vi "LogLabVIEWError.vi"(8 "Error in (no error)":errorcluster, 10 "Error in":errorcluster, 11 "Log in":refnum<class "Log.lvclass">) -> (0 "Error out":errorcluster, 3 "Log out":refnum<class "Log.lvclass">)   [LabVIEW 2011, in "Log.lvclass"]
uses:
  Log.lvclass
  LogCluster.ctl
  PrioritiesRing.ctl
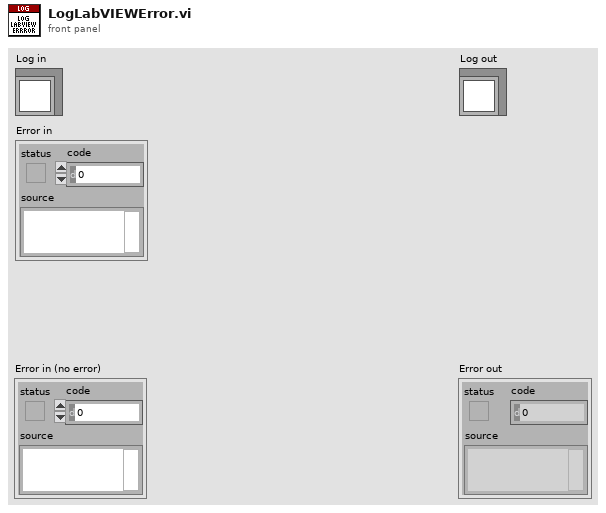
[diagram p1: front panel]
types:
  T1 = typedef "Log.lvclass/LogCluster.ctl" = cluster{"Timestamp":string, "Message":string, "Priority":T2, "PriorityName":string}
  T2 = typedef "Log.lvclass/PrioritiesRing.ctl" = u32
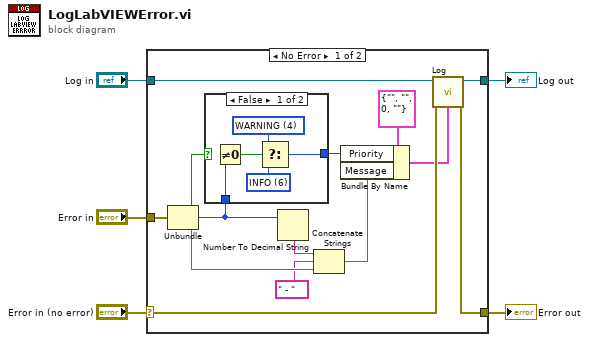
[diagram p0: block diagram]
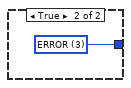
[diagram p2: hidden frame]
diagram:
  n1 = case shown="No Error" "Error in (no error)" {
    selector: "Error in (no error)" -> [w17 w27]
    tunnel: [w16 w27] -> w4
    tunnel: [w18 w26] -> w2
    tunnel: "Log in" -> [w19 w26]
    tunnel: "Error in" -> [w15 _]
    frame No Error {
      n2 = Unbundle(w15) -> ("status"=w11:bool, "code"=w10:i32, "source"=w13:string)
      n3 = case shown="False" w11 {
        tunnel: w10 -> [w20 _]
        tunnel: [w24 w25] -> w8
        frame False {
          w22 = T2 6 items=["EMERGENCY", "ALERT", "CRITICAL", "ERROR", "WARNING", "NOTICE", "INFO", "DEBUG"] ("Ring")
          w21 = T2 4 items=["EMERGENCY", "ALERT", "CRITICAL", "ERROR", "WARNING", "NOTICE", "INFO", "DEBUG"] ("Ring")
          n4 = Not Equal To 0?(x=w20) -> (x != 0?=w23:bool)
          n5 = Select(t=w21, s=w23, f=w22) -> (s? t:f=w24:T2)
        }
        frame True {
          w25 = T2 3 items=["EMERGENCY", "ALERT", "CRITICAL", "ERROR", "WARNING", "NOTICE", "INFO", "DEBUG"] ("Ring")
        }
      }
      n6 = Number To Decimal String(number=w10) -> (decimal integer string=w14:string)  [unwired: 1 in]
      n7 = Concatenate Strings(w14, " - " ("string"), w13) -> (w7:string)
      n8 = Bundle By Name(cluster=T1 {"Timestamp"="", "Message"="", "Priority"=0, "PriorityName"=""} ("Log"), "Priority"=w8, "Message"=w7) -> (w6:T1)
      n9 = call "Log.vi"("Error in (no error)"=w17, 10:"Log in"=w6, 11:"Log in"=w19) -> ("Error out"=w16:errorcluster, "Log out"=w18:refnum<class "Log.lvclass">)  [unwired: 7 in]
    }
    frame Error {
    }
  }
  "Error out" <- w4
  "Log out" <- w2
